vi "EDF-header.vi"(0 "Save channels":i32[](array[numeric])=[0, 1, 2, 3, 4, 5, 6, 7], 1 "Physical minimum":i32[](array[numeric]), 2 "Physical maximum":i32[](array[numeric]), 4 "Physical dimension":string[](array[string])=["mV", "mV", "mV", "mV", "mV", "mV", "mV", "mV", "", "", "", "", "", "", "", "", "", "channel 7", "channel 8"], 5 "Signal labels":string[](array[string])=["channel 1", "channel 2", "channel 3", "channel 4", "channel 5", "channel 6", "channel 7", "channel 8", "", "", "", "", "", "", "", "", "", "channel 7", "channel 8"], 6 "Sample frequency":i32=4096, 9 "Transducer":string[](array[string])=["", "", "", "", "", "", "", "", "", "", "", "", "", "", "", "", "", "channel 7", "channel 8"], 10 "Subject description":string, 11 "Prefilter":string[](array[string])=["", "", "", "", "", "", "", "", "", "", "", "", "", "", "", "", "", "channel 7", "channel 8"], 12 "Digital minimum":i32=-32768, 13 "Digital maximum":i32=32767, 15 "Recording description":string) -> (14 "EDF-header":string)   [LabVIEW 2013]
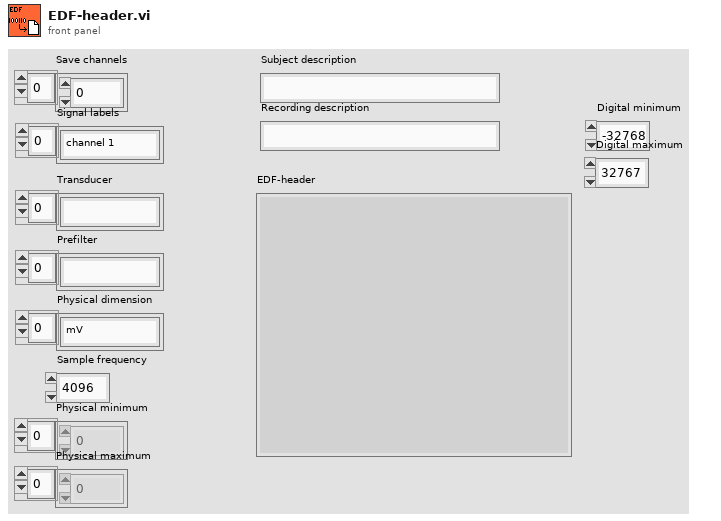
[diagram p1: front panel]
types:
  T1 = cluster{string, string, string, string, string, string, string, string, string, string, string, string, string, string, string, string}
  T2 = cluster{string, string, string, string, string, string}
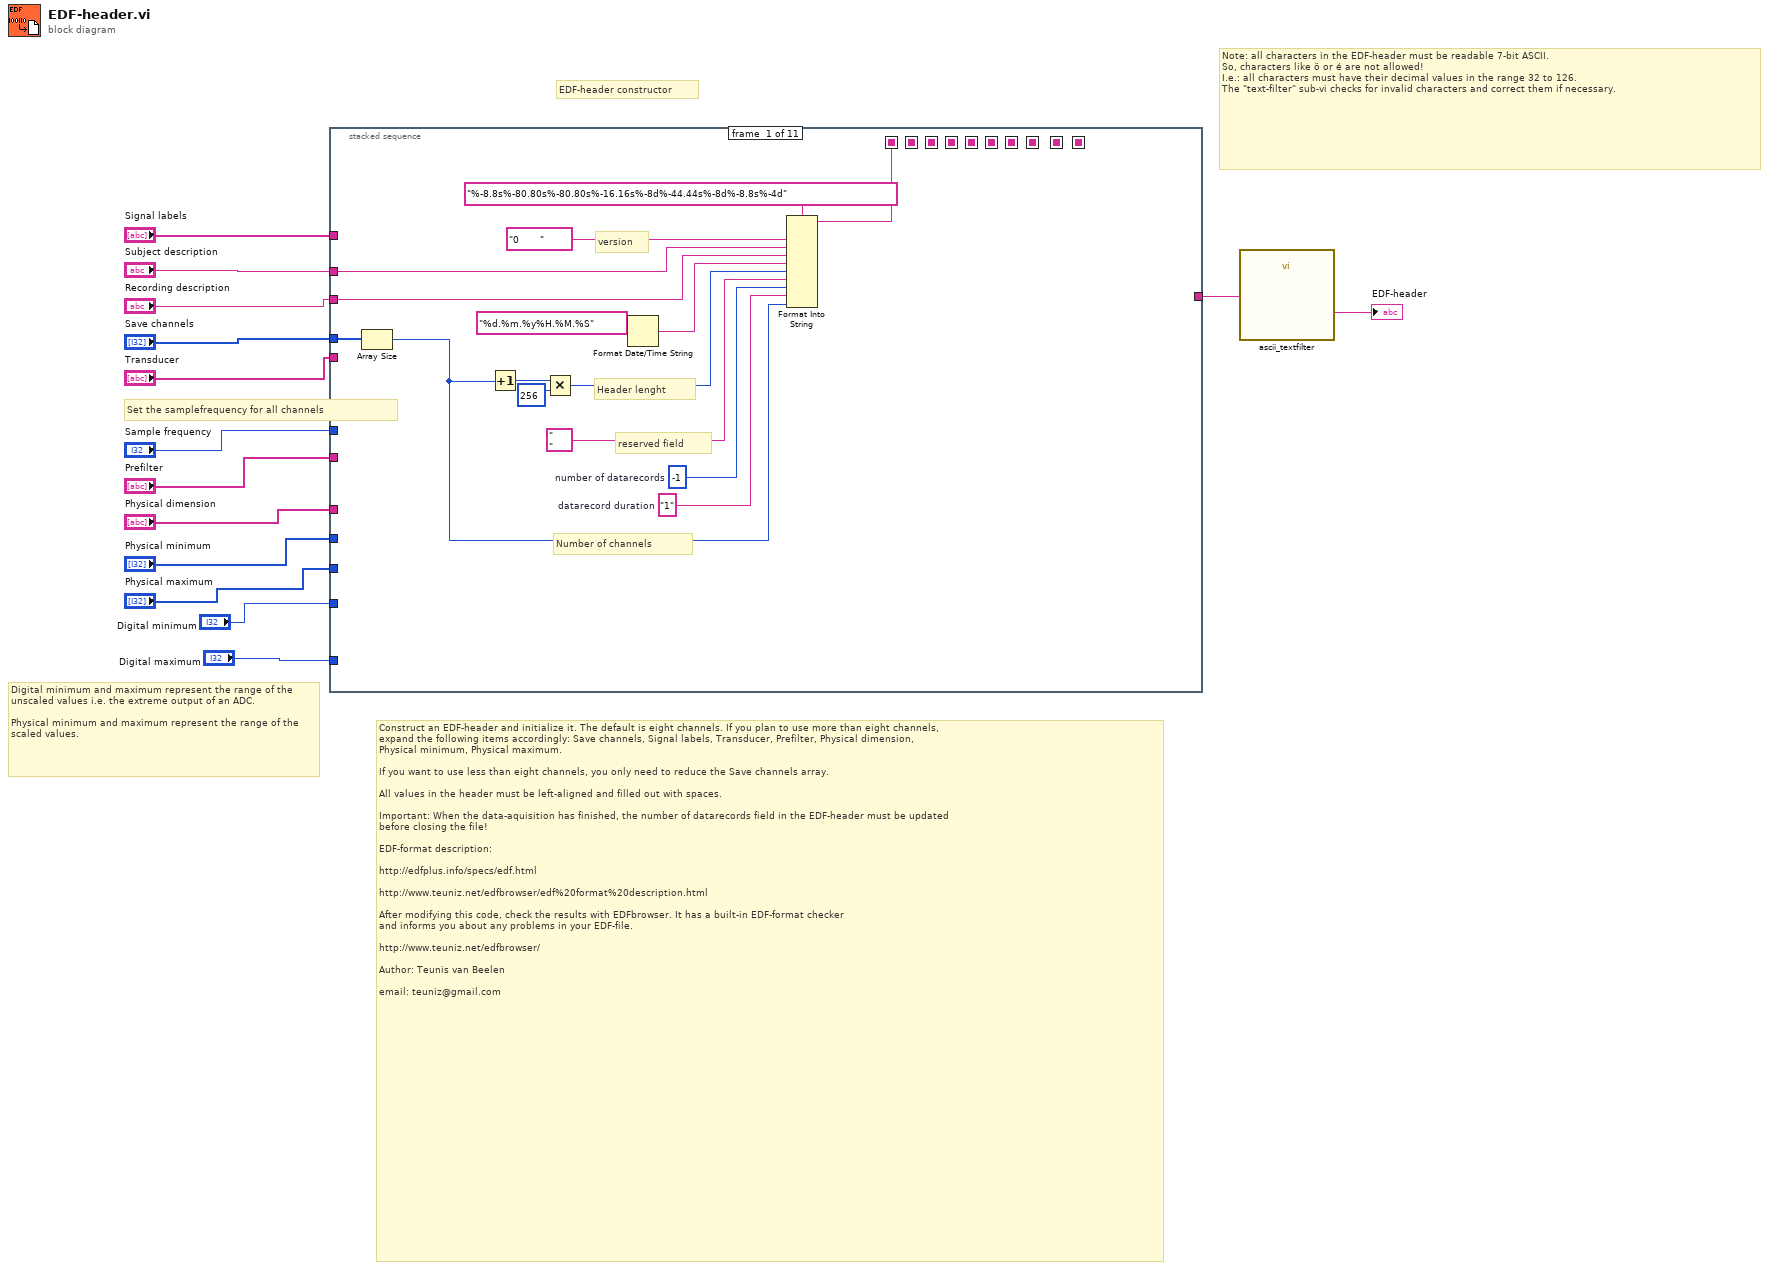
[diagram p0: block diagram]
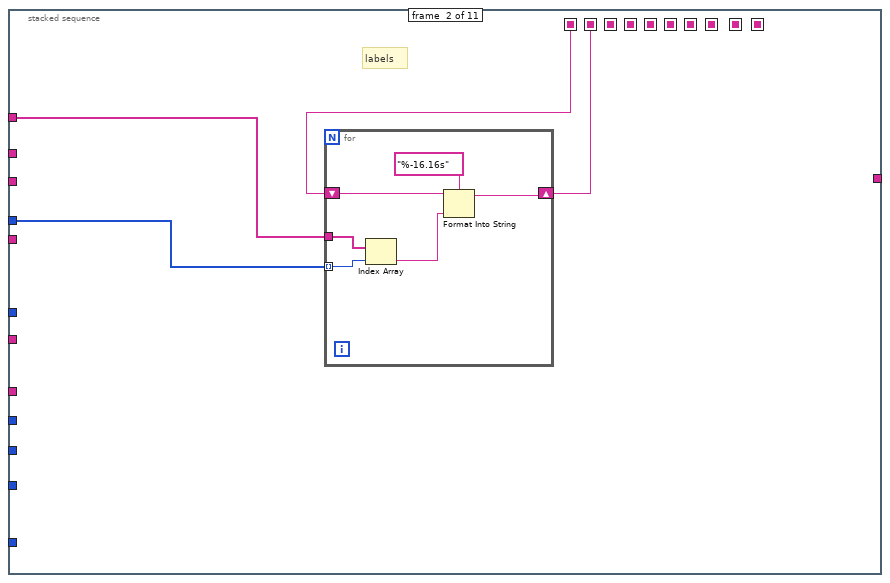
[diagram p2: hidden frame]
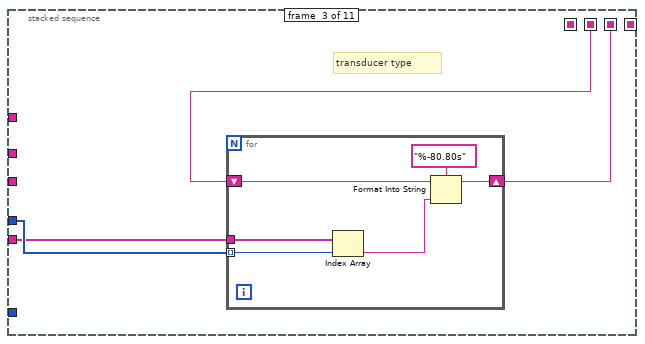
[diagram p3: hidden frame]
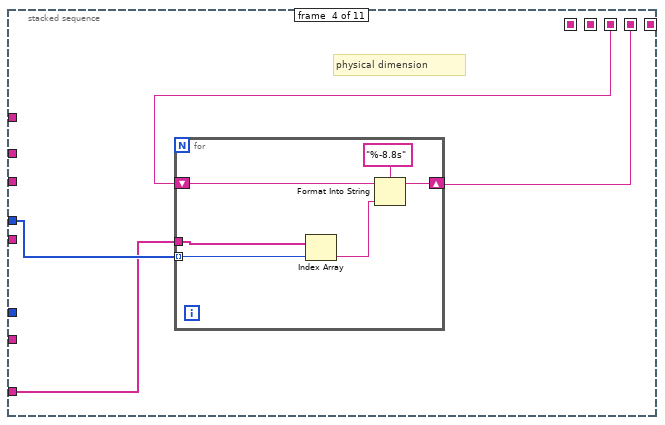
[diagram p4: hidden frame]
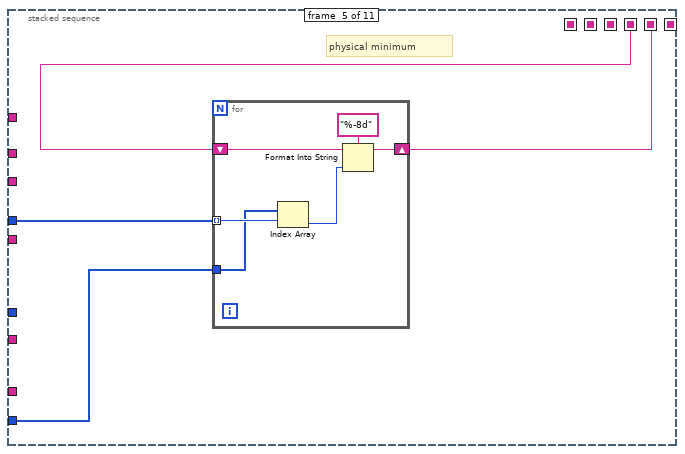
[diagram p5: hidden frame]
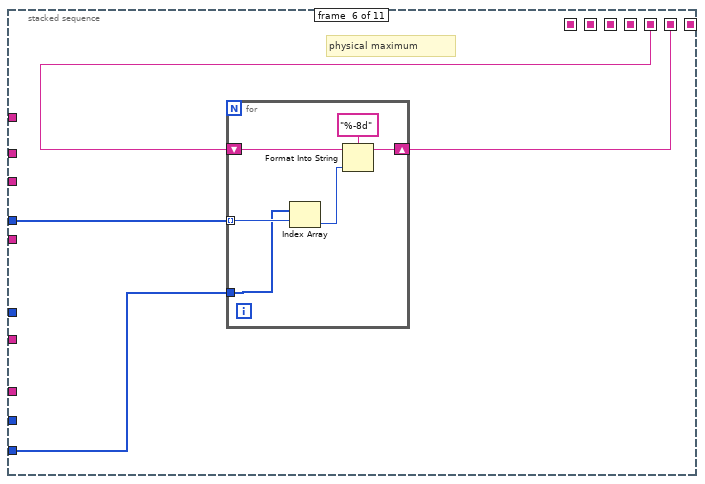
[diagram p6: hidden frame]
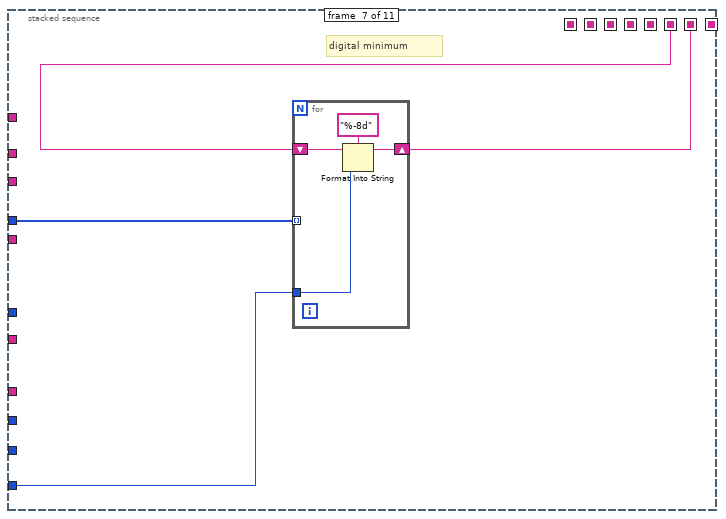
[diagram p7: hidden frame]
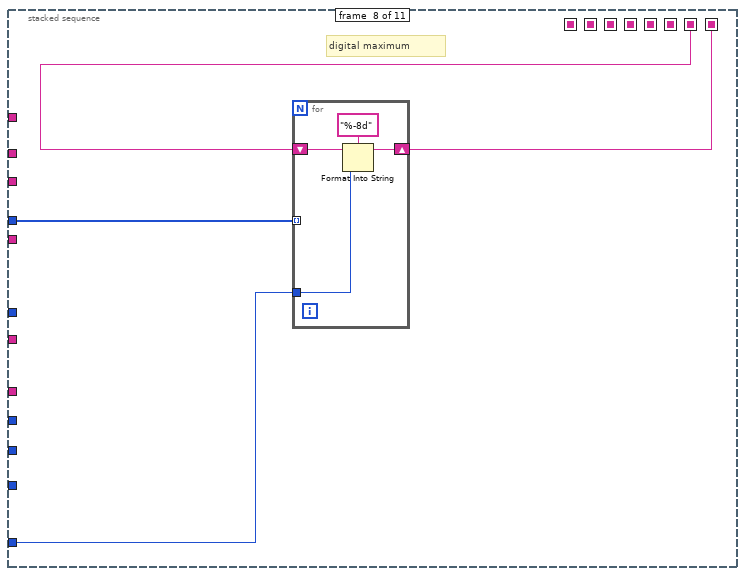
[diagram p8: hidden frame]
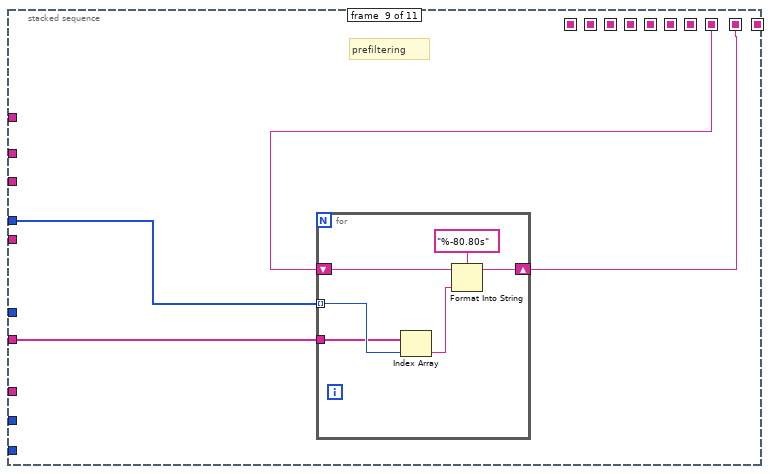
[diagram p9: hidden frame]
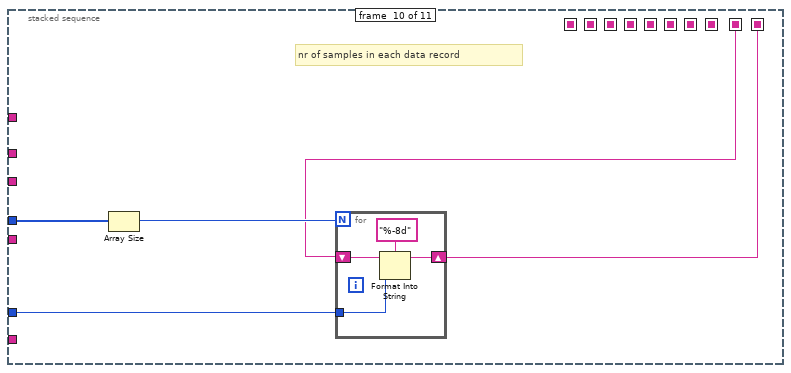
[diagram p10: hidden frame]
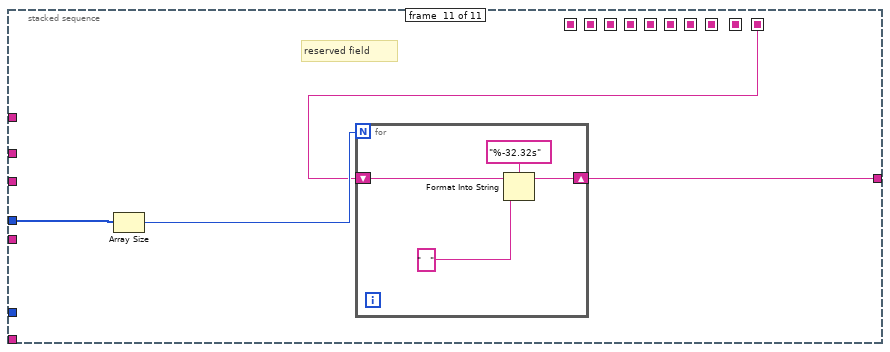
[diagram p11: hidden frame]
diagram:
  # "Digital minimum and maximum represent the range of the unscaled values i.e. the extreme output of an ADC.\n\nPhysical minimum and maximum represent the range of the scaled values."
  # "Note: all characters in the EDF-header must be readable 7-bit ASCII.\nSo, characters like ö or é are not allowed!\nI.e.: all characters must have their decimal values in the range 32 to 126.\nThe \"text-filter\" sub-vi checks for invalid characters and correct them if necessary."
  # "Set the samplefrequency for all channels"
  # "EDF-header constructor"
  # "Construct an EDF-header and initialize it. The default is eight channels. If you plan to use more than eight channels,\nexpand the following items accordingly: Save channels, Signal labels, Transducer, Prefilter, Physical dimension,\nPhysical minimum, Physical maximum.\n\nIf you want to use less than eight channels, you only need to reduce the Save channels array.\n\nAll values in the header must be left-aligned and filled out with spaces.\n\nImportant: When the data-aquisition has finished, the number of datarecords field in the EDF-header must be updated\nbefore closing the file!\n\nEDF-format description:\n\nhttp://edfplus.info/specs/edf.html\n\nhttp://www.teuniz.net/edfbrowser/edf%20format%20description.html\n\nAfter modifying this code, check the results with EDFbrowser. It has a built-in EDF-format checker\nand informs you about any problems in your EDF-file.\n\nhttp://www.teuniz.net/edfbrowser/\n\nAuthor: Teunis van Beelen\n\nemail: teuniz@gmail.com"
  n1 = stacked-sequence {
    seq-local: [w19 _ _ _ _ _ _ _ _ _ _] -> [_ w32 _ _ _ _ _ _ _ _ _]
    seq-local: [_ w30 _ _ _ _ _ _ _ _ _] -> [_ _ w320 _ _ _ _ _ _ _ _]
    seq-local: [_ _ w319 _ _ _ _ _ _ _ _] -> [_ _ _ w330 _ _ _ _ _ _ _]
    seq-local: [_ _ _ w329 _ _ _ _ _ _ _] -> [_ _ _ _ w340 _ _ _ _ _ _]
    seq-local: [_ _ _ _ w339 _ _ _ _ _ _] -> [_ _ _ _ _ w347 _ _ _ _ _]
    seq-local: [_ _ _ _ _ w348 _ _ _ _ _] -> [_ _ _ _ _ _ w357 _ _ _ _]
    seq-local: [_ _ _ _ _ _ w358 _ _ _ _] -> [_ _ _ _ _ _ _ w365 _ _ _]
    seq-local: [_ _ _ _ _ _ _ w366 _ _ _] -> [_ _ _ _ _ _ _ _ w373 _ _]
    seq-local: [_ _ _ _ _ _ _ _ w374 _ _] -> [_ _ _ _ _ _ _ _ _ w384 _]
    seq-local: [_ _ _ _ _ _ _ _ _ w383 _] -> [_ _ _ _ _ _ _ _ _ _ w392]
    tunnel: "Digital minimum" -> [_ _ _ _ _ _ w359 _ _ _ _]
    tunnel: "Digital maximum" -> [_ _ _ _ _ _ _ w367 _ _ _]
    tunnel: "Sample frequency" -> [_ _ _ _ _ _ _ _ _ w387 _]
    tunnel: "Signal labels" -> [_ w31 _ _ _ _ _ _ _ _ _]
    tunnel: "Save channels" -> [w29 w33 w318 w328 w338 w350 w360 w368 w376 w386 w394]
    tunnel: [_ _ _ _ _ _ _ _ _ _ w395] -> w8
    tunnel: "Prefilter" -> [_ _ _ _ _ _ _ _ w375 _ _]
    tunnel: "Transducer" -> [_ _ w317 _ _ _ _ _ _ _ _]
    tunnel: "Physical dimension" -> [_ _ _ w327 _ _ _ _ _ _ _]
    tunnel: "Subject description" -> [w16 _ _ _ _ _ _ _ _ _ _]
    tunnel: "Recording description" -> [w15 _ _ _ _ _ _ _ _ _ _]
    tunnel: "Physical maximum" -> [_ _ _ _ _ w349 _ _ _ _ _]
    tunnel: "Physical minimum" -> [_ _ _ _ w337 _ _ _ _ _ _]
    frame #0 {
      w17 = "1"  # datarecord duration
      w20 = -1  # number of datarecords
      # "version"
      # "reserved field"
      # "Header lenght"
      # "Number of channels"
      n2 = Array Size(array=w29) -> (size(s)=w18:i32)
      n3 = Increment(x=w18) -> (x+1=w23:i32)
      n4 = Multiply(x=w23, y=256 ("x")) -> (x*y=w22:i32)
      n5 = Format Date/Time String(time format string (%c)="%d.%m.%y%H.%M.%S") -> (date/time string=w25:string)  [unwired: 2 in]
      n6 = Format Into String(format string="%-8.8s%-80.80s%-80.80s%-16.16s%-8d%-44.44s%-8d%-8.8s%-4d", "0       ", w16, w15, w25, w22, "     ", w20, w17, w18) -> (resulting string=w19:string)  [unwired: 2 in, 1 out]
    }
    frame #1 {
      (unwired) "%-16.16s%-16.16s%-16.16s%-16.16s%-16.16s%-16.16s%-16.16s%-16.16s%-16.16s%-16.16s%-16.16s%-16.16s%-16.16s%-16.16s%-16.16s%-16.16s%-16.16s%-16.16s%-16.16s%-16.16s%-16.16s%-16.16s%-16.16s%-16.16s%-16.16s%-16.16s%-16.16s%-16.16s%-16.16s%-16.16s%-16.16s%-16.16s%-16.16s%-16.16s%-16.16s%-16.16s%-16.16s%-16.16s%-16.16s%-16.16s%-16.16s%-16.16s%-16.16s%-16.16s%-16.16s%-16.16s%-16.16s%-16.16s%-16.16s%-16.16s%-16.16s%-16.16s%-16.16s%-16.16s%-16.16s%-16.16s%-16.16s%-16.16s%-16.16s%-16.16s%-16.16s%-16.16s%-16.16s%-16.16s%-16.16s%-16.16s%-16.16s%-16.16s%-16.16s%-16.16s%-16.16s%-16.16s%-16.16s%-16.16s%-16.16s%-16.16s%-16.16s%-16.16s%-16.16s%-16.16s%-16.16s%-16.16s%-16.16s%-16.16s%-16.16s%-16.16s%-16.16s%-16.16s%-16.16s%-16.16s%-16.16s%-16.16s%-16.16s%-16.16s%-16.16s%-16.16s%-16.16s%-16.16s%-16.16s%-16.16s%-16.16s%-16.16s%-16.16s%-16.16s%-16.16s%-16.16s%-16.16s%-16.16s%-16.16s%-16.16s%-16.16s%-16.16s%-16.16s%-16.16s%-16.16s%-16.16s%-16.16s%-16.16s%-16.16s%-16.16s%-16.16s%-16.16s%-16.16s%-16.16s%-16.16s%-16.16s%-16.16s%-16.16s%-16.16s%-16.16s%-16.16s%-16.16s%-16.16s%-16.16s"
      (unwired) "%-16.16s%-16.16s%-16.16s%-16.16s%-16.16s%-16.16s%-16.16s%-16.16s%-16.16s%-16.16s%-16.16s%-16.16s%-16.16s%-16.16s%-16.16s%-16.16s%-16.16s%-16.16s%-16.16s%-16.16s%-16.16s%-16.16s%-16.16s%-16.16s%-16.16s%-16.16s%-16.16s%-16.16s%-16.16s%-16.16s%-16.16s%-16.16s%-16.16s%-16.16s%-16.16s%-16.16s%-16.16s%-16.16s%-16.16s%-16.16s%-16.16s%-16.16s%-16.16s%-16.16s%-16.16s%-16.16s%-16.16s%-16.16s%-16.16s%-16.16s%-16.16s%-16.16s%-16.16s%-16.16s%-16.16s%-16.16s%-16.16s%-16.16s%-16.16s%-16.16s%-16.16s%-16.16s%-16.16s%-16.16s%-16.16s%-16.16s%-16.16s%-16.16s%-16.16s%-16.16s%-16.16s%-16.16s%-16.16s%-16.16s%-16.16s%-16.16s%-16.16s%-16.16s%-16.16s%-16.16s%-16.16s%-16.16s%-16.16s%-16.16s%-16.16s%-16.16s%-16.16s%-16.16s%-16.16s%-16.16s%-16.16s%-16.16s%-16.16s%-16.16s%-16.16s%-16.16s%-16.16s%-16.16s%-16.16s%-16.16s%-16.16s%-16.16s%-16.16s%-16.16s%-16.16s%-16.16s%-16.16s%-16.16s%-16.16s%-16.16s%-16.16s%-16.16s%-16.16s%-16.16s%-16.16s%-16.16s%-16.16s%-16.16s%-16.16s%-16.16s%-16.16s%-16.16s%-16.16s%-16.16s%-16.16s%-16.16s%-16.16s%-16.16s%-16.16s%-16.16s%-16.16s%-16.16s%-16.16s%-16.16s"
      # "9"
      # "8"
      # "7"
      # "6"
      # "5"
      # "4"
      # "3"
      # "2"
      # "1"
      # "labels"
      # "9"
      # "8"
      # "7"
      # "6"
      # "5"
      # "4"
      # "3"
      # "2"
      # "1"
      # "134"
      # "9"
      # "8"
      # "7"
      # "6"
      # "5"
      # "4"
      # "3"
      # "2"
      # "1"
      # "label"
      n7 = for {
        tunnel: w33 -> [w315] mode=indexing
        tunnel: w31 -> [w316]
        shift-right: [w314] -> w30
        shift-left: w32 -> [w313]
        n8 = Index Array(array=w316, index=w315) -> (element=w312:string)
        n9 = Format Into String(format string="%-16.16s", initial string=w313, w312) -> (resulting string=w314:string)  [unwired: 1 in, 1 out]
      }
      n10 = Bundle("EEG-001", "EEG-002", "EEG-003", "EEG-004", "EEG-005", "EEG-006", "EEG-007", "EEG-008", "EEG-009", "EEG-010", "EEG-011", "EEG-012", "EEG-013", "EEG-014", "EEG-015", "EEG-016") -> (w294:T1)  [unwired: 1 in]
      n11 = Bundle("EEG-017", "EEG-018", "EEG-019", "EEG-020", "EEG-021", "EEG-022", "EEG-023", "EEG-024", "EEG-025", "EEG-026", "EEG-027", "EEG-028", "EEG-029", "EEG-030", "EEG-031", "EEG-032") -> (w260:T1)  [unwired: 1 in]
      n12 = Bundle("EEG-033", "EEG-034", "EEG-035", "EEG-036", "EEG-037", "EEG-038", "EEG-039", "EEG-040", "EEG-041", "EEG-042", "EEG-043", "EEG-044", "EEG-045", "EEG-046", "EEG-047", "EEG-048") -> (w228:T1)  [unwired: 1 in]
      n13 = Bundle("EEG-049", "EEG-050", "EEG-051", "EEG-052", "EEG-053", "EEG-054", "EEG-055", "EEG-056", "EEG-057", "EEG-058", "EEG-059", "EEG-060", "EEG-061", "EEG-062", "EEG-063", "EEG-064") -> (w195:T1)  [unwired: 1 in]
      n14 = Bundle("EEG-065", "EEG-066", "EEG-067", "EEG-068", "EEG-069", "EEG-070", "EEG-071", "EEG-072", "EEG-073", "EEG-074", "EEG-075", "EEG-076", "EEG-077", "EEG-078", "EEG-079", "EEG-080") -> (w162:T1)  [unwired: 1 in]
      n15 = Bundle("EEG-081", "EEG-082", "EEG-083", "EEG-084", "EEG-085", "EEG-086", "EEG-087", "EEG-088", "EEG-089", "EEG-090", "EEG-091", "EEG-092", "EEG-093", "EEG-094", "EEG-095", "EEG-096") -> (w129:T1)  [unwired: 1 in]
      n16 = Bundle("EEG-097", "EEG-098", "EEG-099", "EEG-100", "EEG-101", "EEG-102", "EEG-103", "EEG-104", "EEG-105", "EEG-106", "EEG-107", "EEG-108", "EEG-109", "EEG-110", "EEG-111", "EEG-112") -> (w112:T1)  [unwired: 1 in]
      n17 = Bundle("EEG-113", "EEG-114", "EEG-115", "EEG-116", "EEG-117", "EEG-118", "EEG-119", "EEG-120", "EEG-121", "EEG-122", "GSR-01", "GSR-02", "GSR-03", "GSR-04", "GSR-05", "GSR-06") -> (w57:T1)  [unwired: 1 in]
      n18 = Bundle("GSR-07", "GSR-08", "GSR-09", "GSR-10", "Respiration", "Status") -> (w56:T2)  [unwired: 1 in]
      n19 = Unbundle(w294) -> (w293:string, w280:string, w279:string, w278:string, w281:string, w282:string, w283:string, w284:string, w285:string, w286:string, w287:string, w288:string, w289:string, w290:string, w291:string, w292:string)
      n20 = Unbundle(w260) -> (w277:string, w259:string, w258:string, w257:string, w256:string, w255:string, w254:string, w253:string, w252:string, w251:string, w250:string, w249:string, w248:string, w247:string, w246:string, w245:string)
      n21 = Unbundle(w228) -> (w227:string, w226:string, w225:string, w224:string, w223:string, w222:string, w221:string, w220:string, w219:string, w218:string, w217:string, w216:string, w215:string, w214:string, w213:string, w212:string)
      n22 = Unbundle(w195) -> (w194:string, w193:string, w192:string, w191:string, w190:string, w189:string, w188:string, w187:string, w186:string, w185:string, w184:string, w183:string, w182:string, w181:string, w180:string, w179:string)
      n23 = Unbundle(w162) -> (w161:string, w160:string, w159:string, w158:string, w157:string, w156:string, w155:string, w154:string, w153:string, w152:string, w151:string, w150:string, w149:string, w148:string, w147:string, w146:string)
      n24 = Unbundle(w129) -> (w111:string, w110:string, w109:string, w108:string, w107:string, w106:string, w105:string, w104:string, w103:string, w102:string, w101:string, w100:string, w99:string, w98:string, w97:string, w96:string)
      n25 = Unbundle(w112) -> (w95:string, w94:string, w93:string, w92:string, w91:string, w90:string, w89:string, w88:string, w87:string, w86:string, w85:string, w84:string, w83:string, w82:string, w81:string, w80:string)
      n26 = Unbundle(w57) -> (w55:string, w54:string, w53:string, w52:string, w51:string, w50:string, w49:string, w48:string, w47:string, w46:string, w45:string, w44:string, w43:string, w42:string, w41:string, w40:string)
      n27 = Unbundle(w56) -> (w39:string, w38:string, w37:string, w36:string, w35:string, w34:string)
      n28 = Format Into String(w293, w280, w279, w278, w281, w282, w283, w284, w285, w286, w287, w288, w289, w290, w291, w292, w277, w259, w258, w257, w256, w255, w254, w253, w252, w251, w250, w249, w248, w247, w246, w245, w227, w226, w225, w224, w223, w222, w221, w220, w219, w218, w217, w216, w215, w214, w213, w212, w194, w193, w192, w191, w190, w189, w188, w187, w186, w185, w184, w183, w182, w181, w180, w179, w161, w160, w159, w158, w157, w156, w155, w154, w153, w152, w151, w150, w149, w148, w147, w146, w111, w110, w109, w108, w107, w106, w105, w104, w103, w102, w101, w100, w99, w98, w97, w96, w95, w94, w93, w92, w91, w90, w89, w88, w87, w86, w85, w84, w83, w82, w81, w80, w55, w54, w53, w52, w51, w50, w49, w48, w47, w46, w45, w44, w43, w42, w41, w40, w39, w38, w37, w36, w35, w34) -> ()  [unwired: 3 in, 2 out]
    }
    frame #2 {
      # "transducer type"
      n29 = for {
        shift-right: [w324] -> w319
        shift-left: w320 -> [w325]
        tunnel: w318 -> [w322] mode=indexing
        tunnel: w317 -> [w321]
        n30 = Index Array(array=w321, index=w322) -> (element=w323:string)
        n31 = Format Into String(format string="%-80.80s" ("Format String"), initial string=w325, w323) -> (resulting string=w324:string)  [unwired: 1 in, 1 out]
      }
    }
    frame #3 {
      # "physical dimension"
      n32 = for {
        shift-right: [w334] -> w329
        shift-left: w330 -> [w335]
        tunnel: w328 -> [w332] mode=indexing
        tunnel: w327 -> [w331]
        n33 = Index Array(array=w331, index=w332) -> (element=w333:string)
        n34 = Format Into String(format string="%-8.8s" ("Format String"), initial string=w335, w333) -> (resulting string=w334:string)  [unwired: 1 in, 1 out]
      }
    }
    frame #4 {
      # "physical minimum"
      n35 = for {
        shift-right: [w344] -> w339
        shift-left: w340 -> [w345]
        tunnel: w338 -> [w343] mode=indexing
        tunnel: w337 -> [w341]
        n36 = Index Array(array=w341, index=w343) -> (element=w342:i32)
        n37 = Format Into String(format string="%-8d" ("Format String"), initial string=w345, w342) -> (resulting string=w344:string)  [unwired: 1 in, 1 out]
      }
    }
    frame #5 {
      # "physical maximum"
      n38 = for {
        shift-right: [w354] -> w348
        shift-left: w347 -> [w355]
        tunnel: w349 -> [w352]
        tunnel: w350 -> [w353] mode=indexing
        n39 = Index Array(array=w352, index=w353) -> (element=w351:i32)
        n40 = Format Into String(format string="%-8d" ("Format String"), initial string=w355, w351) -> (resulting string=w354:string)  [unwired: 1 in, 1 out]
      }
    }
    frame #6 {
      # "digital minimum"
      n41 = for {
        shift-right: [w361] -> w358
        shift-left: w357 -> [w362]
        tunnel: w359 -> [w363]
        tunnel: w360 -> [_] mode=indexing
        n42 = Format Into String(format string="%-8d" ("Format String"), initial string=w362, w363) -> (resulting string=w361:string)  [unwired: 1 in, 1 out]
      }
    }
    frame #7 {
      # "digital maximum"
      n43 = for {
        shift-right: [w369] -> w366
        shift-left: w365 -> [w370]
        tunnel: w367 -> [w371]
        tunnel: w368 -> [_] mode=indexing
        n44 = Format Into String(format string="%-8d" ("Format String"), initial string=w370, w371) -> (resulting string=w369:string)  [unwired: 1 in, 1 out]
      }
    }
    frame #8 {
      # "prefiltering"
      n45 = for {
        shift-right: [w380] -> w374
        shift-left: w373 -> [w381]
        tunnel: w376 -> [w379] mode=indexing
        tunnel: w375 -> [w377]
        n46 = Index Array(array=w377, index=w379) -> (element=w378:string)
        n47 = Format Into String(format string="%-80.80s" ("Format String"), initial string=w381, w378) -> (resulting string=w380:string)  [unwired: 1 in, 1 out]
      }
    }
    frame #9 {
      # "nr of samples in each data record"
      n48 = Array Size(array=w386) -> (size(s)=w385:i32)
      n49 = for {
        N: w385 -> [_]
        tunnel: w387 -> [w391]
        shift-right: [w388] -> w383
        shift-left: w384 -> [w389]
        n50 = Format Into String(format string="%-8d" ("Format String"), initial string=w389, w391) -> (resulting string=w388:string)  [unwired: 1 in, 1 out]
      }
    }
    frame #10 {
      # "reserved field"
      n51 = Array Size(array=w394) -> (size(s)=w393:i32)
      n52 = for {
        N: w393 -> [_]
        shift-right: [w396] -> w395
        shift-left: w392 -> [w397]
        n53 = Format Into String(format string="%-32.32s" ("Format String"), initial string=w397, "   ") -> (resulting string=w396:string)  [unwired: 1 in, 1 out]
      }
    }
  }
  n54 = call "ascii_textfilter.vi"("Inputstring"=w8) -> ("Outputstring"=→"EDF-header":string)  [unwired: 10 in]
